vi "OtherInfo.vi"(0 "refnum":refnum<file>, 11 "offset":i32) -> (4 "dup refnum":refnum<file>, 6 "comment":string, 8 "filler":string)   [LabVIEW 2022 SP3]
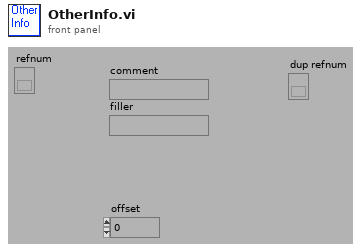
[diagram p1: front panel]
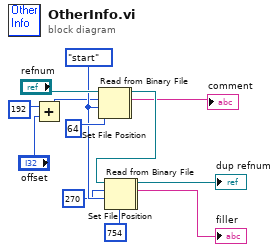
[diagram p0: block diagram]
diagram:
  w9 = enum16{"start", "end", "current"}."start" ("pos mode (0:2)")
  n1 = Add(x=192 ("pos offset (0)"), y="offset") -> (x+y=w7:i32)
  n2 = Set File Position(offset (in bytes) (0)=w7, refnum="refnum", from (0:start)=w9) -> (refnum out=w2:refnum<file>, error out=w1:errorcluster)  [unwired: 1 in]
  n3 = Read from Binary File(8:w1, 10:64 ("count"), 11:w2) -> (2:→"comment":string, 3:w13:refnum<file>)  [unwired: 5 out]
  n4 = Set File Position(offset (in bytes) (0)=270 ("pos offset (0)"), refnum=w13, from (0:start)=w9) -> (refnum out=w4:refnum<file>, error out=w3:errorcluster)  [unwired: 1 in]
  n5 = Read from Binary File(8:w3, 10:754 ("count"), 11:w4) -> (2:→"filler":string, 3:→"dup refnum":refnum<file>)  [unwired: 5 out]
